vi "dynamika.vi"(2 "error in":errorcluster, 3 "dynamika [nm/s]":dbl(slide)=400.0 scale=0.0..1000.0, 4 "scansize [nm]":dbl(slide)=1.0 scale=0.0..5000.0) -> (0 "error out":errorcluster, 1 "czas trwania [s]":dbl)   [LabVIEW 2013]
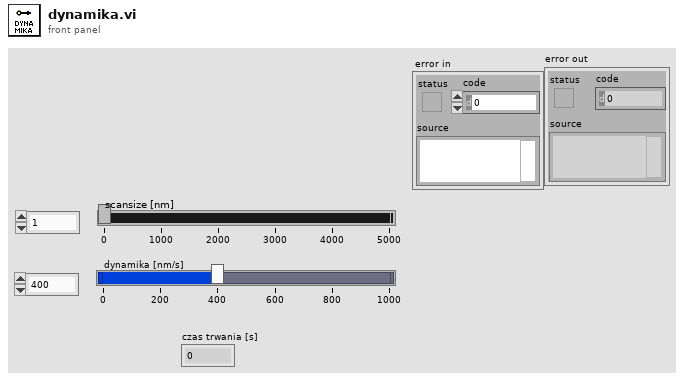
[diagram p1: front panel]
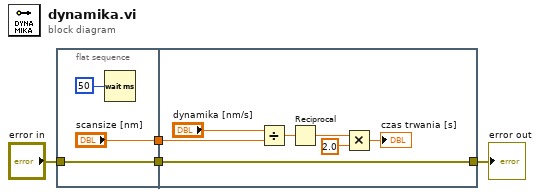
[diagram p0: block diagram]
diagram:
  n1 = flat-sequence {
    tunnel: ["scansize [nm]"] -> w4
    tunnel: [w5] -> w3
    tunnel: "error in" -> [w5]
    tunnel: w4 -> [w13]
    tunnel: w3 -> [w11]
    tunnel: [w11] -> w1
    frame #0 {
      n2 = Wait (ms)(milliseconds to wait=u32 50) -> ()  [unwired: 1 out]
    }
    frame #1 {
      n3 = Divide(x="dynamika [nm/s]", y=w13) -> (x/y=w14:dbl)
      n4 = Reciprocal(x=w14) -> (1/x=w8:dbl)
      n5 = Multiply(x=w8, y=2.0 ("1/x")) -> (x*y=→"czas trwania [s]":dbl)
    }
  }
  "error out" <- w1
